vi "仪器运行状态读取.vi"(4 "error in (no error)":errorcluster caption="错误输入（无错误）", 6 "Container State":T7 caption="容器状态", 7 "Display State In":T1={"配置信息"={"周期模式"=enum."不启用", "定点周期"={"启动命令"=0, "启动命令 2"=0, "启动命令 3"=0, "启动命令 4"=0, "启动命令 5"=0, "启动命令 6"=0, "启动命令 7"=0, "启动命令 8"=0, "启动命令 9"=0, "启动命令 10"=0, "启动命令 11"=0, "启动命令 12"=0, "启动命令 13"=0, "启动命令 14"=0, "启动命令 15"=0, "启动命令 16"=0, "启动命令 17"=0, "启动命令 18"=0, "启动命令 19"=0, "启动命令 20"=0, "启动命令 21"=0, "启动命令 22"=0, "启动命令 23"=0, "启动命令 24"=0}, "间隔启动"={"启动命令"=0, "启动间隔"=0.0, "启动次数"=0}, "测量参数"={"氨氮"=TRUE, "总磷"=TRUE, "总氮"=TRUE, "CODMn"=TRUE, "CODCr"=TRUE}}, "仪器运行状态"=FALSE, "启动次数"=0, "最近一次启动时间"=timestamp(0 s since 1904-01-01), "最近一次结束时间"=timestamp(0 s since 1904-01-01), "间隔计时"=0.0, "时间源"={"时间源选择"=enum."系统时间源", "外部时间源"=timestamp(0 s since 1904-01-01)}, "引用参数"=""} caption="显示状态输入" {"配置信息"."间隔启动"."启动命令" items=["", "加标回收（启动采配水）", "加标回收（不启动采配水）", "水样测试（启动采配水）", "水样测试（不启动采配水）"]; "配置信息"."定点周期"."启动命令 24" items=["", "加标回收（启动采配水）", "加标回收（不启动采配水）", "水样测试（启动采配水）", "水样测试（不启动采配水）"]; "配置信息"."定点周期"."启动命令 23" items=["", "加标回收（启动采配水）", "加标回收（不启动采配水）", "水样测试（启动采配水）", "水样测试（不启动采配水）"]; "配置信息"."定点周期"."启动命令 22" items=["", "加标回收（启动采配水）", "加标回收（不启动采配水）", "水样测试（启动采配水）", "水样测试（不启动采配水）"]; "配置信息"."定点周期"."启动命令 21" items=["", "加标回收（启动采配水）", "加标回收（不启动采配水）", "水样测试（启动采配水）", "水样测试（不启动采配水）"]; "配置信息"."定点周期"."启动命令 20" items=["", "加标回收（启动采配水）", "加标回收（不启动采配水）", "水样测试（启动采配水）", "水样测试（不启动采配水）"]; "配置信息"."定点周期"."启动命令 19" items=["", "加标回收（启动采配水）", "加标回收（不启动采配水）", "水样测试（启动采配水）", "水样测试（不启动采配水）"]; "配置信息"."定点周期"."启动命令 18" items=["", "加标回收（启动采配水）", "加标回收（不启动采配水）", "水样测试（启动采配水）", "水样测试（不启动采配水）"]; "配置信息"."定点周期"."启动命令 17" items=["", "加标回收（启动采配水）", "加标回收（不启动采配水）", "水样测试（启动采配水）", "水样测试（不启动采配水）"]; "配置信息"."定点周期"."启动命令 16" items=["", "加标回收（启动采配水）", "加标回收（不启动采配水）", "水样测试（启动采配水）", "水样测试（不启动采配水）"]; "配置信息"."定点周期"."启动命令 15" items=["", "加标回收（启动采配水）", "加标回收（不启动采配水）", "水样测试（启动采配水）", "水样测试（不启动采配水）"]; "配置信息"."定点周期"."启动命令 14" items=["", "加标回收（启动采配水）", "加标回收（不启动采配水）", "水样测试（启动采配水）", "水样测试（不启动采配水）"]; "配置信息"."定点周期"."启动命令 13" items=["", "加标回收（启动采配水）", "加标回收（不启动采配水）", "水样测试（启动采配水）", "水样测试（不启动采配水）"]; "配置信息"."定点周期"."启动命令 12" items=["", "加标回收（启动采配水）", "加标回收（不启动采配水）", "水样测试（启动采配水）", "水样测试（不启动采配水）"]; "配置信息"."定点周期"."启动命令 11" items=["", "加标回收（启动采配水）", "加标回收（不启动采配水）", "水样测试（启动采配水）", "水样测试（不启动采配水）"]; "配置信息"."定点周期"."启动命令 10" items=["", "加标回收（启动采配水）", "加标回收（不启动采配水）", "水样测试（启动采配水）", "水样测试（不启动采配水）"]; "配置信息"."定点周期"."启动命令 9" items=["", "加标回收（启动采配水）", "加标回收（不启动采配水）", "水样测试（启动采配水）", "水样测试（不启动采配水）"]; "配置信息"."定点周期"."启动命令 8" items=["", "加标回收（启动采配水）", "加标回收（不启动采配水）", "水样测试（启动采配水）", "水样测试（不启动采配水）"]; "配置信息"."定点周期"."启动命令 7" items=["", "加标回收（启动采配水）", "加标回收（不启动采配水）", "水样测试（启动采配水）", "水样测试（不启动采配水）"]; "配置信息"."定点周期"."启动命令 6" items=["", "加标回收（启动采配水）", "加标回收（不启动采配水）", "水样测试（启动采配水）", "水样测试（不启动采配水）"]; "配置信息"."定点周期"."启动命令 5" items=["", "加标回收（启动采配水）", "加标回收（不启动采配水）", "水样测试（启动采配水）", "水样测试（不启动采配水）"]; "配置信息"."定点周期"."启动命令 4" items=["", "加标回收（启动采配水）", "加标回收（不启动采配水）", "水样测试（启动采配水）", "水样测试（不启动采配水）"]; "配置信息"."定点周期"."启动命令 3" items=["", "加标回收（启动采配水）", "加标回收（不启动采配水）", "水样测试（启动采配水）", "水样测试（不启动采配水）"]; "配置信息"."定点周期"."启动命令 2" items=["", "加标回收（启动采配水）", "加标回收（不启动采配水）", "水样测试（启动采配水）", "水样测试（不启动采配水）"]; "配置信息"."定点周期"."启动命令" items=["", "加标回收（启动采配水）", "加标回收（不启动采配水）", "水样测试（启动采配水）", "水样测试（不启动采配水）"]}) -> (0 "error out":errorcluster caption="错误输出", 2 "Value":bool caption="值", 3 "Display State Out":T1={"配置信息"={"周期模式"=enum."不启用", "定点周期"={"启动命令"=0, "启动命令 2"=0, "启动命令 3"=0, "启动命令 4"=0, "启动命令 5"=0, "启动命令 6"=0, "启动命令 7"=0, "启动命令 8"=0, "启动命令 9"=0, "启动命令 10"=0, "启动命令 11"=0, "启动命令 12"=0, "启动命令 13"=0, "启动命令 14"=0, "启动命令 15"=0, "启动命令 16"=0, "启动命令 17"=0, "启动命令 18"=0, "启动命令 19"=0, "启动命令 20"=0, "启动命令 21"=0, "启动命令 22"=0, "启动命令 23"=0, "启动命令 24"=0}, "间隔启动"={"启动命令"=0, "启动间隔"=0.0, "启动次数"=0}, "测量参数"={"氨氮"=TRUE, "总磷"=TRUE, "总氮"=TRUE, "CODMn"=TRUE, "CODCr"=TRUE}}, "仪器运行状态"=FALSE, "启动次数"=0, "最近一次启动时间"=timestamp(0 s since 1904-01-01), "最近一次结束时间"=timestamp(0 s since 1904-01-01), "间隔计时"=0.0, "时间源"={"时间源选择"=enum."系统时间源", "外部时间源"=timestamp(0 s since 1904-01-01)}, "引用参数"=""} caption="显示状态输出" {"配置信息"."间隔启动"."启动命令" items=["", "加标回收（启动采配水）", "加标回收（不启动采配水）", "水样测试（启动采配水）", "水样测试（不启动采配水）"]; "配置信息"."定点周期"."启动命令 24" items=["", "加标回收（启动采配水）", "加标回收（不启动采配水）", "水样测试（启动采配水）", "水样测试（不启动采配水）"]; "配置信息"."定点周期"."启动命令 23" items=["", "加标回收（启动采配水）", "加标回收（不启动采配水）", "水样测试（启动采配水）", "水样测试（不启动采配水）"]; "配置信息"."定点周期"."启动命令 22" items=["", "加标回收（启动采配水）", "加标回收（不启动采配水）", "水样测试（启动采配水）", "水样测试（不启动采配水）"]; "配置信息"."定点周期"."启动命令 21" items=["", "加标回收（启动采配水）", "加标回收（不启动采配水）", "水样测试（启动采配水）", "水样测试（不启动采配水）"]; "配置信息"."定点周期"."启动命令 20" items=["", "加标回收（启动采配水）", "加标回收（不启动采配水）", "水样测试（启动采配水）", "水样测试（不启动采配水）"]; "配置信息"."定点周期"."启动命令 19" items=["", "加标回收（启动采配水）", "加标回收（不启动采配水）", "水样测试（启动采配水）", "水样测试（不启动采配水）"]; "配置信息"."定点周期"."启动命令 18" items=["", "加标回收（启动采配水）", "加标回收（不启动采配水）", "水样测试（启动采配水）", "水样测试（不启动采配水）"]; "配置信息"."定点周期"."启动命令 17" items=["", "加标回收（启动采配水）", "加标回收（不启动采配水）", "水样测试（启动采配水）", "水样测试（不启动采配水）"]; "配置信息"."定点周期"."启动命令 16" items=["", "加标回收（启动采配水）", "加标回收（不启动采配水）", "水样测试（启动采配水）", "水样测试（不启动采配水）"]; "配置信息"."定点周期"."启动命令 15" items=["", "加标回收（启动采配水）", "加标回收（不启动采配水）", "水样测试（启动采配水）", "水样测试（不启动采配水）"]; "配置信息"."定点周期"."启动命令 14" items=["", "加标回收（启动采配水）", "加标回收（不启动采配水）", "水样测试（启动采配水）", "水样测试（不启动采配水）"]; "配置信息"."定点周期"."启动命令 13" items=["", "加标回收（启动采配水）", "加标回收（不启动采配水）", "水样测试（启动采配水）", "水样测试（不启动采配水）"]; "配置信息"."定点周期"."启动命令 12" items=["", "加标回收（启动采配水）", "加标回收（不启动采配水）", "水样测试（启动采配水）", "水样测试（不启动采配水）"]; "配置信息"."定点周期"."启动命令 11" items=["", "加标回收（启动采配水）", "加标回收（不启动采配水）", "水样测试（启动采配水）", "水样测试（不启动采配水）"]; "配置信息"."定点周期"."启动命令 10" items=["", "加标回收（启动采配水）", "加标回收（不启动采配水）", "水样测试（启动采配水）", "水样测试（不启动采配水）"]; "配置信息"."定点周期"."启动命令 9" items=["", "加标回收（启动采配水）", "加标回收（不启动采配水）", "水样测试（启动采配水）", "水样测试（不启动采配水）"]; "配置信息"."定点周期"."启动命令 8" items=["", "加标回收（启动采配水）", "加标回收（不启动采配水）", "水样测试（启动采配水）", "水样测试（不启动采配水）"]; "配置信息"."定点周期"."启动命令 7" items=["", "加标回收（启动采配水）", "加标回收（不启动采配水）", "水样测试（启动采配水）", "水样测试（不启动采配水）"]; "配置信息"."定点周期"."启动命令 6" items=["", "加标回收（启动采配水）", "加标回收（不启动采配水）", "水样测试（启动采配水）", "水样测试（不启动采配水）"]; "配置信息"."定点周期"."启动命令 5" items=["", "加标回收（启动采配水）", "加标回收（不启动采配水）", "水样测试（启动采配水）", "水样测试（不启动采配水）"]; "配置信息"."定点周期"."启动命令 4" items=["", "加标回收（启动采配水）", "加标回收（不启动采配水）", "水样测试（启动采配水）", "水样测试（不启动采配水）"]; "配置信息"."定点周期"."启动命令 3" items=["", "加标回收（启动采配水）", "加标回收（不启动采配水）", "水样测试（启动采配水）", "水样测试（不启动采配水）"]; "配置信息"."定点周期"."启动命令 2" items=["", "加标回收（启动采配水）", "加标回收（不启动采配水）", "水样测试（启动采配水）", "水样测试（不启动采配水）"]; "配置信息"."定点周期"."启动命令" items=["", "加标回收（启动采配水）", "加标回收（不启动采配水）", "水样测试（启动采配水）", "水样测试（不启动采配水）"]})   [LabVIEW 2016, in "ZK定时设置.xctl"]
uses:
  <vilib>/_xctls/Container State.ctl
  <vilib>/_xctls/XControlSupport.lvlib
panel:
  # "将以下值显示控件替换为所需类型的显示控件。\n不要从连线板中删除该显示控件或其它显示控件。\n不要更改连线板模式。\n值显示控件应始终位于连线板输出端自顶部起第二个接线端。"
  # "分钟"
  # "次"
  # "分钟"
  # "次"
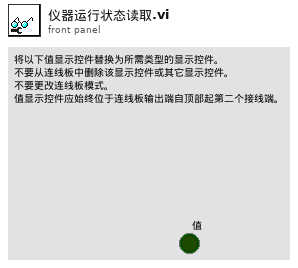
[diagram p1: front panel]
types:
  T1 = typedef "ZK定时设置.xctl/状态.ctl" = cluster{"配置信息":cluster{"周期模式":T2, "定点周期":T3, "间隔启动":T5, "测量参数":T6}, "仪器运行状态":bool, "启动次数":i32, "最近一次启动时间":timestamp, "最近一次结束时间":timestamp, "间隔计时":dbl, "时间源":cluster{"时间源选择":enum16{"系统时间源", "仪器时间源"}, "外部时间源":timestamp}, "引用参数":string}
  T2 = typedef "ZK定时设置.xctl/周期模式设置.ctl" = enum16{"不启用", "定点模式", "间隔模式"}
  T3 = typedef "ZK定时设置.xctl/定点周期设置.ctl" = cluster{"启动命令":T4, "启动命令 2":T4, "启动命令 3":T4, "启动命令 4":T4, "启动命令 5":T4, "启动命令 6":T4, "启动命令 7":T4, "启动命令 8":T4, "启动命令 9":T4, "启动命令 10":T4, "启动命令 11":T4, "启动命令 12":T4, "启动命令 13":T4, "启动命令 14":T4, "启动命令 15":T4, "启动命令 16":T4, "启动命令 17":T4, "启动命令 18":T4, "启动命令 19":T4, "启动命令 20":T4, "启动命令 21":T4, "启动命令 22":T4, "启动命令 23":T4, "启动命令 24":T4}
  T4 = typedef "ZK定时设置.xctl/启动命令选择.ctl" = u16
  T5 = typedef "ZK定时设置.xctl/间隔启动设置.ctl" = cluster{"启动命令":T4, "启动间隔":dbl, "启动次数":i32}
  T6 = typedef "ZK定时设置.xctl/测量参数.ctl" = cluster{"氨氮":bool, "总磷":bool, "总氮":bool, "CODMn":bool, "CODCr":bool}
  T7 = typedef "XControlSupport.lvlib/Container State.ctl" = cluster{"Indicator?":bool, "Run Mode?":bool, " Refnum":refnum<vi>}
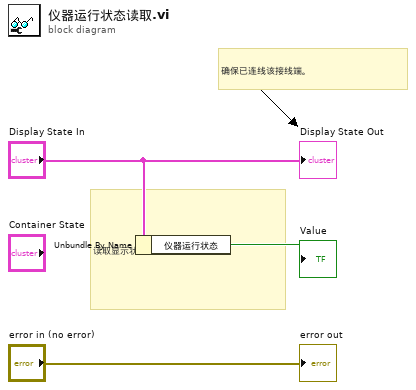
[diagram p0: block diagram]
diagram:
  # "确保已连线该接线端。"
  # "读取显示状态并更新属性值。"
  n1 = Unbundle By Name("Display State In") -> ("仪器运行状态"=→"Value":bool)
  "error out" <- "error in (no error)"
  "Display State Out" <- "Display State In"
